vi "Execution_Appli_SetupGenericSettings.vi"(8 "error in":errorcluster, 11 "EVE in":refnum<class "EVE.lvclass">) -> (0 "error out":errorcluster, 3 "EVE out":refnum<class "EVE.lvclass">)   [LabVIEW 2013, in "EVE.lvclass"]
uses:
  EVE.lvclass
  EVE.lvclass/EVE.ctl
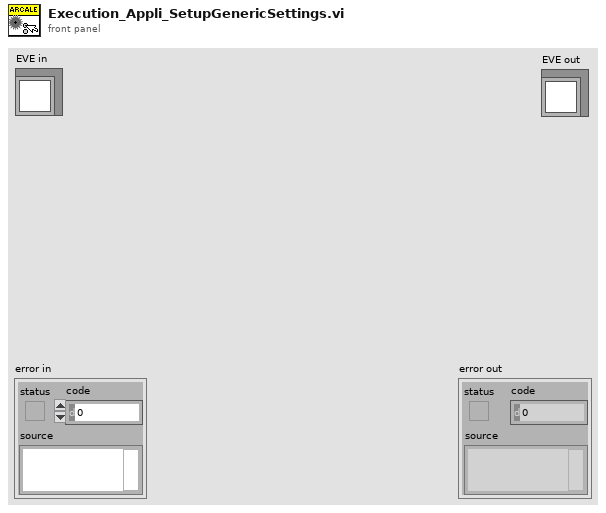
[diagram p1: front panel]
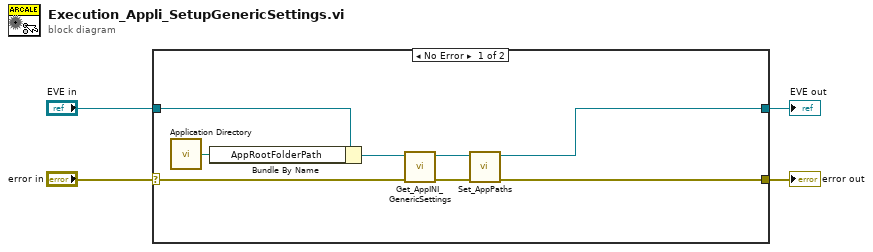
[diagram p0: block diagram]
diagram:
  n1 = case shown="No Error" "error in" {
    selector: "error in" -> [w6 w14]
    tunnel: [w5 w14] -> w3
    tunnel: [w12 w13] -> w1
    tunnel: "EVE in" -> [w9 w13]
    frame No Error {
      n2 = call <vilib>:"Application Directory.vi"() -> ("Application Directory"=w10:path)
      n3 = Bundle By Name(cluster=w9, "AppRootFolderPath"=w10) -> (w11:refnum<class "EVE.lvclass">)
      n4 = call "Get_AppINI_GenericSettings.vi"("error in (no error)"=w6, "EVE in"=w11) -> ("error out"=w7:errorcluster, "EVE out"=w8:refnum<class "EVE.lvclass">)  [unwired: 8 in]
      n5 = call-dynamic "Set_AppPaths.vi"("error in"=w7, "EVE in"=w8) -> ("error out"=w5:errorcluster, "EVE out"=w12:refnum<class "EVE.lvclass">)  [unwired: 8 in]
    }
    frame Error {
    }
  }
  "error out" <- w3
  "EVE out" <- w1
